vi "check range.vi"(6 "lower limit":i32, 7 "upper limit":i32, 8 "error in (no error)":errorcluster, 11 "Mapping":u16) -> (0 "error out":errorcluster)   [LabVIEW 2019, in "Modbus Master System Explorer.lvlib"]
uses:
  Modbus Master System Explorer.lvlib
  <vilib>/ErrorRing/Error Ring.xnode
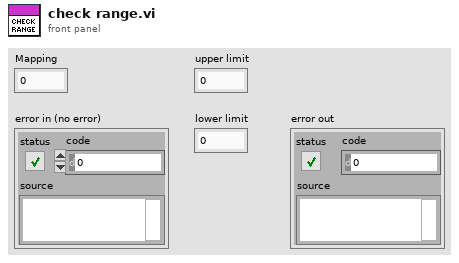
[diagram p1: front panel]
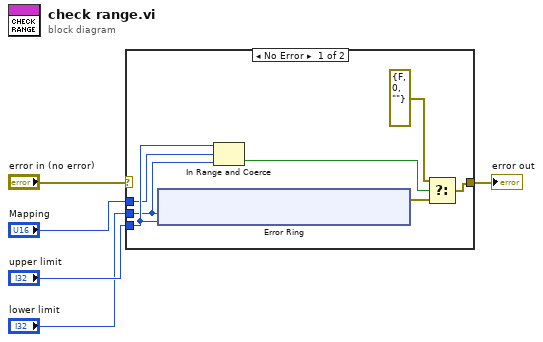
[diagram p0: block diagram]
diagram:
  n1 = case shown="No Error" "error in (no error)" {
    selector: "error in (no error)" -> [_ w19]
    tunnel: [w12 w19] -> w5
    tunnel: "upper limit" -> [w9 _]
    tunnel: "lower limit" -> [w8 _]
    tunnel: "Mapping" -> [w6 _]
    frame No Error {
      n2 = xnode "Error Ring"("parameter 0"=w8, "parameter 1"=w9) -> ("error out"=w10:errorcluster)
      n3 = In Range and Coerce(upper limit=w9, x=w6, lower limit=w8) -> (In Range?=w7:bool)  [unwired: 1 out]
      n4 = Select(t=errorcluster {"status"=FALSE, "code"=0, "source"=""}, s=w7, f=w10) -> (s? t:f=w12:errorcluster)
    }
    frame Error {
    }
  }
  "error out" <- w5
